vi "ToolsPanelPan.vi"(8 "error in (no error)":errorcluster caption="entrée d'erreur (pas d'erreur)", 11 "SR530.lvclass":refnum<class "SR530.lvclass">) -> (0 "error out":errorcluster caption="sortie d'erreur", 3 "SR530.lvclass Out":refnum<class "SR530.lvclass">)   [LabVIEW 2019, in "SR530.lvclass"]
uses:
  SR530.lvclass
  C:/Programmes LabView/LabScanV1A/DevicesClass/BaseDevice/BaseDevice.lvclass
  <userlib>/SR530/Inputs.ctl
  BaseDevice/Accessor/GetClassEvent.vi
panel:
  in  "Output":u16(ring) items=["X5", "X6"]
  in  "Input":u16(ring) items=["X1", "X2", "X3", "X4"]
  in  "Acq":bool
  out "RefFreq":dbl=1000.0 caption="Ref Freq (Hz)" min=0.0 step=0.1 format="%#_5f"
  in  "AnalogOutX":dbl=1000.0 caption="Analog Out X (V)" min=0.0 step=0.1 format="%^#_6e"
  out "AnalogInX":dbl=1000.0 caption="Analog In X (V)" min=0.0 step=0.1 format="%^#_6e"
  in  "Stop":bool
  out "Init Program":bool
  in  "Update":bool caption="stopSpectro"
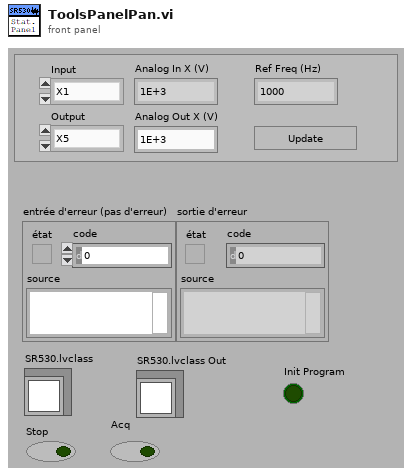
[diagram p1: front panel]
types:
  T1 = enum8{"Enabled", "Disabled", "Disabled and Grayed Out"}
  T2 = cluster{"Channel":u16, "Outputs":dbl[], "Status Byte":bool[]}
  T3 = typedef "Inputs.ctl" = u16
  T4 = cluster{"BandFilter":bool, "LineFilter1x":bool, "LineFilter2x":bool, "Expand Ch1":bool, "Expand Ch2":bool, "Sensitivity":u16, "Pre Time":u16, "Post Time":u16, "Dynamic Res.":u16, "Reference Trigger":u16, "Channels Settings":u16, "Frequency":dbl}
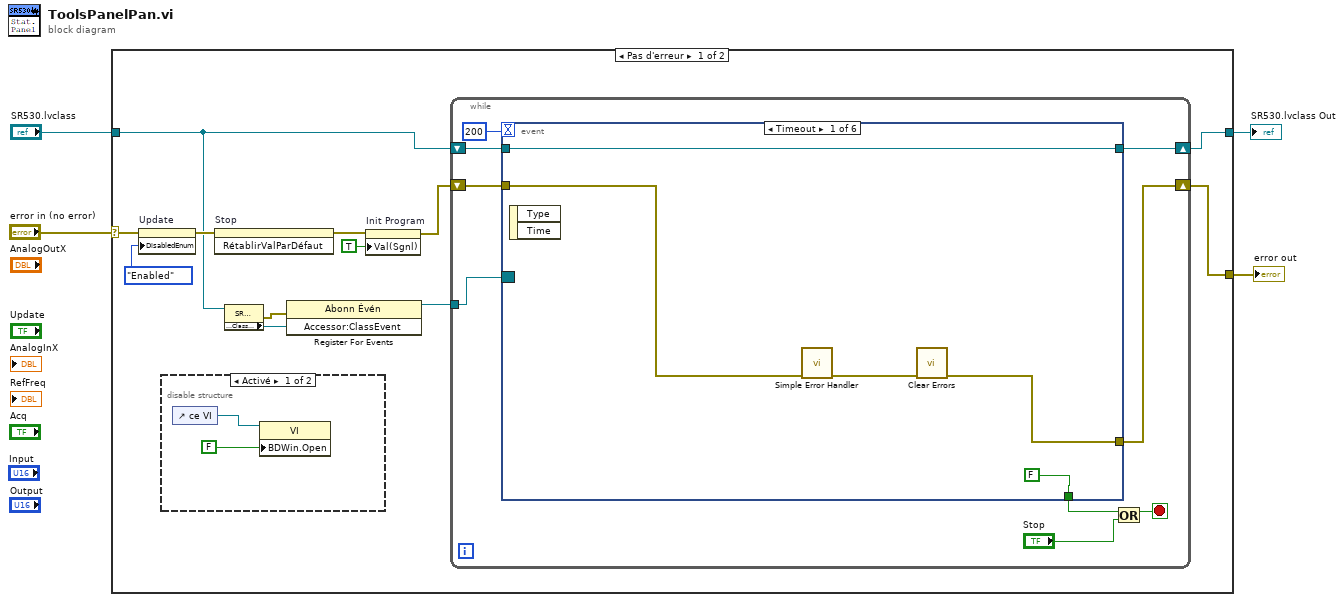
[diagram p0: block diagram]
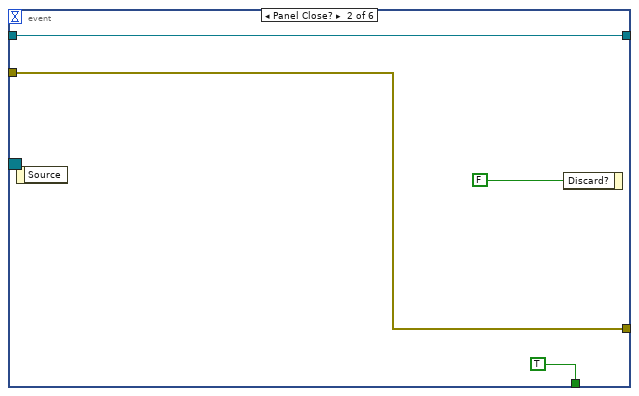
[diagram p3: hidden frame]
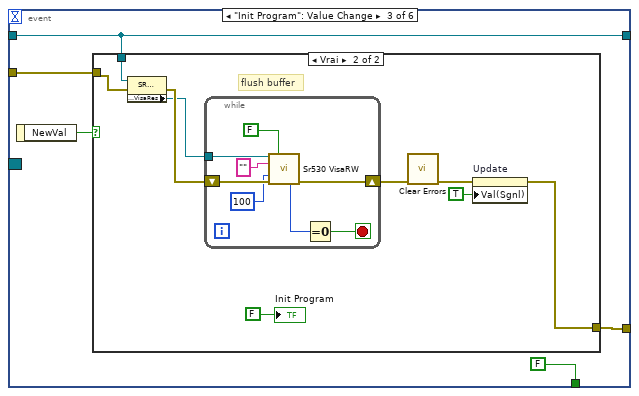
[diagram p4: hidden frame]
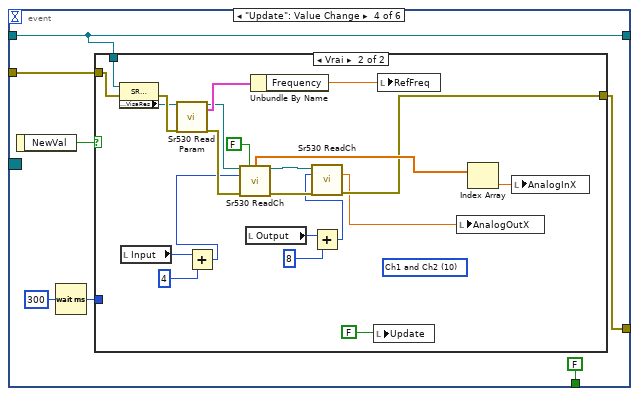
[diagram p6: hidden frame]
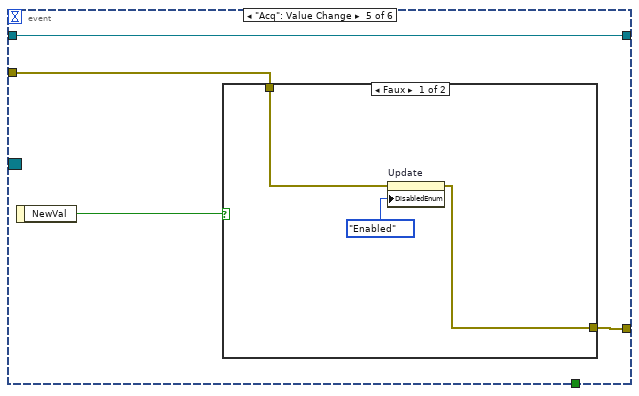
[diagram p8: hidden frame]
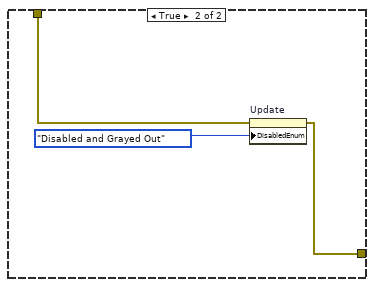
[diagram p9: hidden frame]
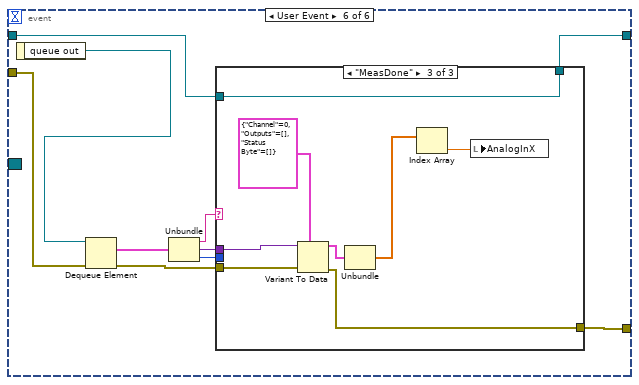
[diagram p10: hidden frame]
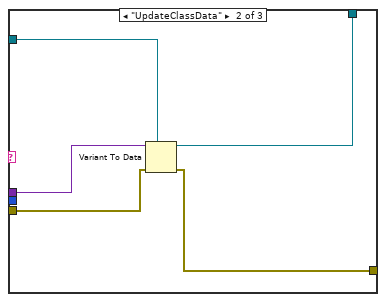
[diagram p12: hidden frame]
diagram:
  n1 = case shown="Pas d'erreur" "error in (no error)" {
    selector: "error in (no error)" -> [w12 w126]
    tunnel: [w5 w126] -> w3
    tunnel: "SR530.lvclass" -> [w6 w125]
    tunnel: [w15 w125] -> w1
    frame No Error {
      n2 = property on="Update" class="Bool (strict)"(error in=w12, "DisabledEnum"=T1."Enabled" ("Désactivé")) -> (error out=w9:errorcluster)  [unwired: 1 in, 1 out]
      n3 = disable-structure shown="Activé" {
        frame Enabled {
          n4 = control-ref of="ce VI"() -> (w18:refnum<vi>)
          n5 = property class="VI"(reference=w18, "BDWin.Open"=FALSE ("Fenêtre du diagramme : ouverte")) -> ()  [unwired: 1 in, 2 out]
        }
        frame Disabled {
        }
      }
      n6 = invoke on="Stop" class="Bool (strict)" method="RétablirValParDéfaut"(error in=w9) -> (error out=w14:errorcluster)  [unwired: 2 in, 2 out]
      n7 = property class="SR530.lvclass"(reference=w6) -> (error out=w10:errorcluster, "Accessor:ClassEvent"=w11:refnum<user-event>)  [unwired: 1 in, 1 out]
      n8 = register-events(error in=w10, w11) -> (reference out=w8:refnum<event-registration>)  [unwired: 1 in, 1 out]
      n9 = property on="Init Program" class="Bool (strict)"(error in=w14, "Val(Sgnl)"=TRUE ("Valeur (Signalisation)")) -> (error out=w7:errorcluster)  [unwired: 1 in, 1 out]
      n10 = while {
        shift-right: [w25] -> w5
        shift-left: w7 -> [w26]
        shift-right: [w22] -> w15
        shift-left: w6 -> [w24]
        tunnel: w8 -> [w19]
        stop <- w21 stop-if-true
        n11 = event shown="[0] Timeout" {
          selector: w19 -> [_ _ _ _ _ _]
          dyn-events: _ -> [_ _ _ _ _ _]
          timeout: 200 -> [_ _ _ _ _ _]
          tunnel: w26 -> [w30 w34 w40 w60 w93 w107]
          tunnel: [w28 w34 w39 w65 w91 w100] -> w25
          tunnel: w24 -> [w31 w33 w37 w61 w90 w103]
          tunnel: [FALSE TRUE FALSE FALSE _ _] -> w23
          tunnel: [w31 w33 w37 w61 w90 w102] -> w22
          event Timeout {
            n12 = event-data() -> ()  [unwired: 1 in, 2 out]
            n13 = call <vilib>:"Simple Error Handler.vi"("error in (no error)"=w30) -> ("error out"=w29:errorcluster)  [unwired: 4 in, 4 out]
            n14 = call <vilib>:"Clear Errors.vi"("error in (no error)"=w29) -> ("error out"=w28:errorcluster)  [unwired: 5 in, 1 out]
          }
          event Panel Close? {
            n15 = event-data() -> ()  [unwired: 1 in, 1 out]
            n16 = event-data("Discard?"=FALSE ("Rejeter ?")) -> ()  [unwired: 1 in, 1 out]
          }
          event "Init Program": Value Change {
            n17 = event-data() -> ("NewVal"=w41:bool)  [unwired: 1 in]
            n18 = case shown="Vrai" w41 {
              tunnel: w40 -> [w42 w47]
              tunnel: [w42 w49] -> w39
              tunnel: w37 -> [_ w46]
              frame False {
              }
              frame True {
                # "flush buffer"
                n19 = property class="SR530.lvclass"(reference=w46, error in=w47) -> (error out=w45:errorcluster, "Accessor:VisaRes"=w44:refnum<visa-resource-name>)  [unwired: 1 out]
                n20 = while {
                  tunnel: w44 -> [w58]
                  shift-right: [w54] -> w48
                  shift-left: w45 -> [w59]
                  stop <- w52 stop-if-true
                  n21 = call <userlib>:"Sr530 VisaRW.vi"("VISA Rsrc"=w58, "2Lecture?"=FALSE, "ChaineCom"="", "Nbcaract"=u32 100, "error in (no error)"=w59) -> ("Count out"=w53:u32, "error out"=w54:errorcluster)  [unwired: 5 in, 4 out]
                  n22 = Equal To 0?(x=w53) -> (x = 0?=w52:bool)
                }
                n23 = call <vilib>:"Clear Errors.vi"("error in (no error)"=w48) -> ("error out"=w43:errorcluster)  [unwired: 5 in, 1 out]
                n24 = property on="Update" class="Bool (strict)"(error in=w43, "Val(Sgnl)"=TRUE ("Valeur (Signalisation)")) -> (error out=w49:errorcluster)  [unwired: 1 in, 1 out]
                "Init Program" <- FALSE
              }
            }
          }
          event "Update": Value Change {
            n25 = event-data() -> ("NewVal"=w66:bool)  [unwired: 1 in]
            n26 = Wait (ms)(milliseconds to wait=u32 300 ("attente (ms)")) -> (millisecond timer value=w62:u32)
            n27 = case shown="Vrai" w66 {
              tunnel: w60 -> [w67 w82]
              tunnel: [w67 w69] -> w65
              tunnel: w62 -> [_ _]
              tunnel: w61 -> [_ w85]
              frame False {
              }
              frame True {
                (unwired) T3 10 items=["Channel 1", "X Output", "Channel 2", "Y Output", "X1", "X2", "X3", "X4", "X5", "X6", "Ch1 and Ch2", "X and Y", "X,Y,Ch1,Ch2"] ("Channel")
                n28 = property class="SR530.lvclass"(reference=w85, error in=w82) -> (error out=w84:errorcluster, "Accessor:VisaRes"=w83:refnum<visa-resource-name>)  [unwired: 1 out]
                n29 = local read "Input"() -> (w77:u16)
                n30 = call <userlib>:"Sr530 Read Param.vi"("Ressource VISA"=w83, "error in (no error)"=w84) -> ("Ressource VISA Out"=w80:refnum<visa-resource-name>, "LockInPar"=w88:T4, "error out"=w81:errorcluster)  [unwired: 14 in, 1 out]
                n31 = Add(x=w77, y=u16 4) -> (x+y=w75:u16)
                n32 = call <userlib>:"Sr530 ReadCh.vi"("VISA Rsrc"=w80, "Autoscale"=FALSE, "Channel"=w75, "error in (no error)"=w81) -> ("Outputs"=w78:dbl[], "Ressource VISA Out"=w73:refnum<visa-resource-name>, "error out"=w74:errorcluster)  [unwired: 4 in, 5 out]
                n33 = local read "Output"() -> (w71:u16)
                n34 = Unbundle By Name(w88) -> ("Frequency"=w87:dbl)
                n35 = Add(x=w71, y=u16 8) -> (x+y=w70:u16)
                n36 = call <userlib>:"Sr530 ReadCh.vi"("VISA Rsrc"=w73, "Channel"=w70, "error in (no error)"=w74) -> ("Output"=w68:dbl, "error out"=w69:errorcluster)  [unwired: 5 in, 6 out]
                n37 = local write "Update"(FALSE) -> ()
                n38 = local write "RefFreq"(w87) -> ()
                n39 = local write "AnalogOutX"(w68) -> ()
                n40 = Index Array(array=w78) -> (element=w89:dbl)  [unwired: 1 in]
                n41 = local write "AnalogInX"(w89) -> ()
              }
            }
          }
          event "Acq": Value Change {
            n42 = event-data() -> ("NewVal"=w92:bool)  [unwired: 1 in]
            n43 = case shown="Faux" w92 {
              tunnel: w93 -> [w95 w98]
              tunnel: [w94 w97] -> w91
              frame False {
                n44 = property on="Update" class="Bool (strict)"(error in=w95, "DisabledEnum"=T1."Enabled" ("Désactivé")) -> (error out=w94:errorcluster)  [unwired: 1 in, 1 out]
              }
              frame True {
                n45 = property on="Update" class="Bool (strict)"(error in=w98, "DisabledEnum"=T1."Disabled and Grayed Out" ("Désactivé")) -> (error out=w97:errorcluster)  [unwired: 1 in, 1 out]
              }
            }
          }
          event User Event {
            n46 = event-data() -> ("queue out"=w108:refnum<queue>)  [unwired: 1 in]
            n47 = Dequeue Element(queue=w108, error in (no error)=w107) -> (element=w109:cluster{"Message":string, "Data":variant, i32}, error out=w101:errorcluster)  [unwired: 1 in, 2 out]
            n48 = Unbundle(w109) -> ("Message"=w106:string, "Data"=w105:variant, w104:i32)
            n49 = case shown="\"MeasDone\"" w106 {
              tunnel: w105 -> [_ w114 w123]
              tunnel: w104 -> [_ _ _]
              tunnel: w103 -> [w111 w116 w124]
              tunnel: [w111 w115 w124] -> w102
              tunnel: w101 -> [w110 w113 w122]
              tunnel: [w110 w112 w121] -> w100
              frame Default {
              }
              frame "UpdateClassData" {
                n50 = Variant To Data(error in=w113, type=w116, Variant=w114) -> (data=w115:refnum<class "SR530.lvclass">, error out=w112:errorcluster)
              }
              frame "MeasDone" {
                n51 = Variant To Data(error in=w122, type=T2 {"Channel"=0, "Outputs"=[], "Status Byte"=[]} ("cluster"), Variant=w123) -> (data=w120:T2, error out=w121:errorcluster)
                n52 = Unbundle(w120) -> ("Outputs"=w118:dbl[])  [unwired: 2 out]
                n53 = Index Array(array=w118) -> (element=w117:dbl)  [unwired: 1 in]
                n54 = local write "AnalogInX"(w117) -> ()
              }
            }
          }
        }
        n55 = Or(x=w23, y="Stop") -> (x .or. y?=w21:bool)
      }
    }
    frame Error {
    }
  }
  "error out" <- w3
  "SR530.lvclass Out" <- w1
